vi "XY_LockMotors_CT.vi"() -> (2 "Command":string)   [LabVIEW 2017]
uses:
  sobot structures/SoBot_CommandTypes.ctl
  sobot structures/XY_Commands.ctl
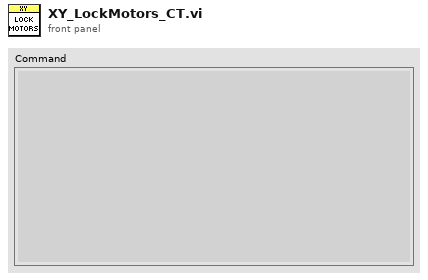
[diagram p1: front panel]
types:
  T1 = typedef "XY_Commands.ctl" = enum16{"XY_Initialize", "XY_MoveToPosition", "XY_MarkTarget", "XY_LockMotors", "XY_UnlockMotors"}
  T2 = typedef "SoBot_CommandTypes.ctl" = enum16{"General_Command", "XY_Command", "Z_Command", "Plattform_Command"}
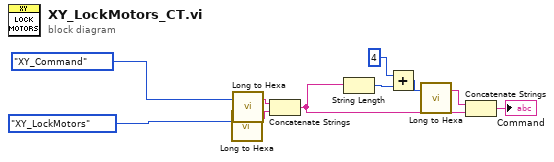
[diagram p0: block diagram]
diagram:
  n1 = call "Long to Hexa.vi"("Long"=XY_Commands."XY_LockMotors" ("XY_Command")) -> ("Hexa"=w9:string)  [unwired: 2 in]
  n2 = call "Long to Hexa.vi"("Long"=SoBot_CommandTypes."XY_Command" ("SoBot_CommandTypes")) -> ("Hexa"=w10:string)  [unwired: 2 in]
  n3 = Concatenate Strings(w10, w9) -> (w4:string)
  n4 = String Length(string=w4) -> (length=w8:i32)
  n5 = Add(x=4, y=w8) -> (x+y=w6:i32)
  n6 = call "Long to Hexa.vi"("Long"=w6) -> ("Hexa"=w5:string)  [unwired: 2 in]
  n7 = Concatenate Strings(w5, w4) -> (→"Command":string)
